vi "DAQ.vi"() -> ()   [LabVIEW 2018]
uses:
  <vilib>/Simulation/DiscreteLinear/Implementation/NILVSim Discrete Transfer Function Direct.llb/SIM Discrete Transfer Function Diagram (SISO CD).vi
  <vilib>/Simulation/ContinuousLinear/Implementation/Shared/SIM Transfer Function Support.llb/SIM Convert CD TF to SIM (SISO).vi
  <vilib>/Simulation/ContinuousLinear/Implementation/Shared/SIM Transfer Function Support.llb/SIM TransferFunction Normalize to Buffer.vi
  <vilib>/Simulation/DiscreteLinear/Implementation/Shared/SIM Init Discrete States.vi
  <vilib>/Simulation/DiscreteLinear/Implementation/NILVSim Discrete Transfer Function Direct.llb/SIM Transfer Function Direct core (SISO).vi
  <vilib>/Simulation/ContinuousLinear/Implementation/Shared/SIM Transfer Function Support.llb/SIM TransferFunction Normalize.vi
  <vilib>/Simulation/Implementation/Shared/SIM Polynomials.llb/SIM Remove Zero Coefficients (DBL).vi
  <vilib>/addons/Control Design/_Model Construction/Model Creation.llb/Model Creation SubVI/cd_Create Transfer Function Model.vi
  <vilib>/addons/Control Design/_Time Response Analysis/Time Response.llb/Time Response subVI/cd_Step Response (Transfer Function).vi
  <vilib>/addons/Control Design/_Utility/Model Viewer.llb/Model Viewer SubVI/cd_Draw Transfer Function Equation (TF).vi
  <vilib>/addons/Control Design/_Model Conversions/Continuous and Discrete.llb/Continuous and Discrete SubVI/cd_Convert Continuous to Discrete (TF).vi
  <vilib>/Simulation/Implementation/Shared/SIM Polynomials.llb/SIM Divide Polynomials (DBL).vi
  <vilib>/Simulation/Implementation/Shared/SIM BuildSimErr.vi
  <vilib>/addons/control/pid/pid.llb/PID (DBL).vi
  <vilib>/Simulation/Implementation/XNodeFramework/SimXNode/SimX.xnode
  <vilib>/addons/Control Design/_Model Construction/Model Typedefs.llb/CD Transfer Function Model (MIMO).ctl
  <vilib>/addons/Control Design/_Model Construction/Model Typedefs.llb/CD General Elements.ctl
  <vilib>/addons/Control Design/_Model Construction/Model Typedefs.llb/CD Transfer Function Model (SISO).ctl
  <vilib>/addons/Control Design/_Model Conversions/NI_CD_Continuous and Discrete.lvlib
  <vilib>/addons/Control Design/_Model Construction/NI_LinSys_Model Typedefs.lvlib
  <vilib>/addons/control/pid/NI_PID_pid.lvlib
  <vilib>/addons/Control Design/_Model Construction/NI_LinSys_Model Creation.lvlib
  <vilib>/addons/Control Design/_Utility/NI_CD_Model Viewer.lvlib
  <vilib>/addons/Control Design/_Time Response Analysis/NI_CD_Time Response.lvlib
  <vilib>/Analysis/NI_AALPro.lvlib
panel:
  in  "Plant Control":i32(knob) scale=0.0..1.0
  out "Step Response\nGraph":cluster{"time":dbl[], dbl[]}[](graph)
  out "Transfer Function Equation":picture
  in  "Sampling\nTime":dbl
  in  "Blower Opening Control at Plant":dbl(slide) scale=15.0..90.0
  out "Polynomial Fit (Fixed)\nfor Temp-Voltage":i32=2
  in  "Voltage input":dbl(knob) scale=0.0..10.0
  in  "Set Temperature\n Auto Mode":i32(slide) scale=20.0..90.0
  in  "output range":cluster{"output high":dbl, "output low":dbl}
  out "Set Temperature Value":dbl
  in  "PID Gains":T1={"proportional gain (Kc)"=1.0, "integral time (Ti, min)"=0.01, "derivative time (Td, min)"=0.0} {"derivative time (Td, min)" format="%.3f"; "integral time (Ti, min)" format="%.3f"; "proportional gain (Kc)" format="%.3f"}
  out "Voltage vs Time":dbl(graph)
  out "Temperature vs Time":dbl(graph)
  in  "STOP":bool
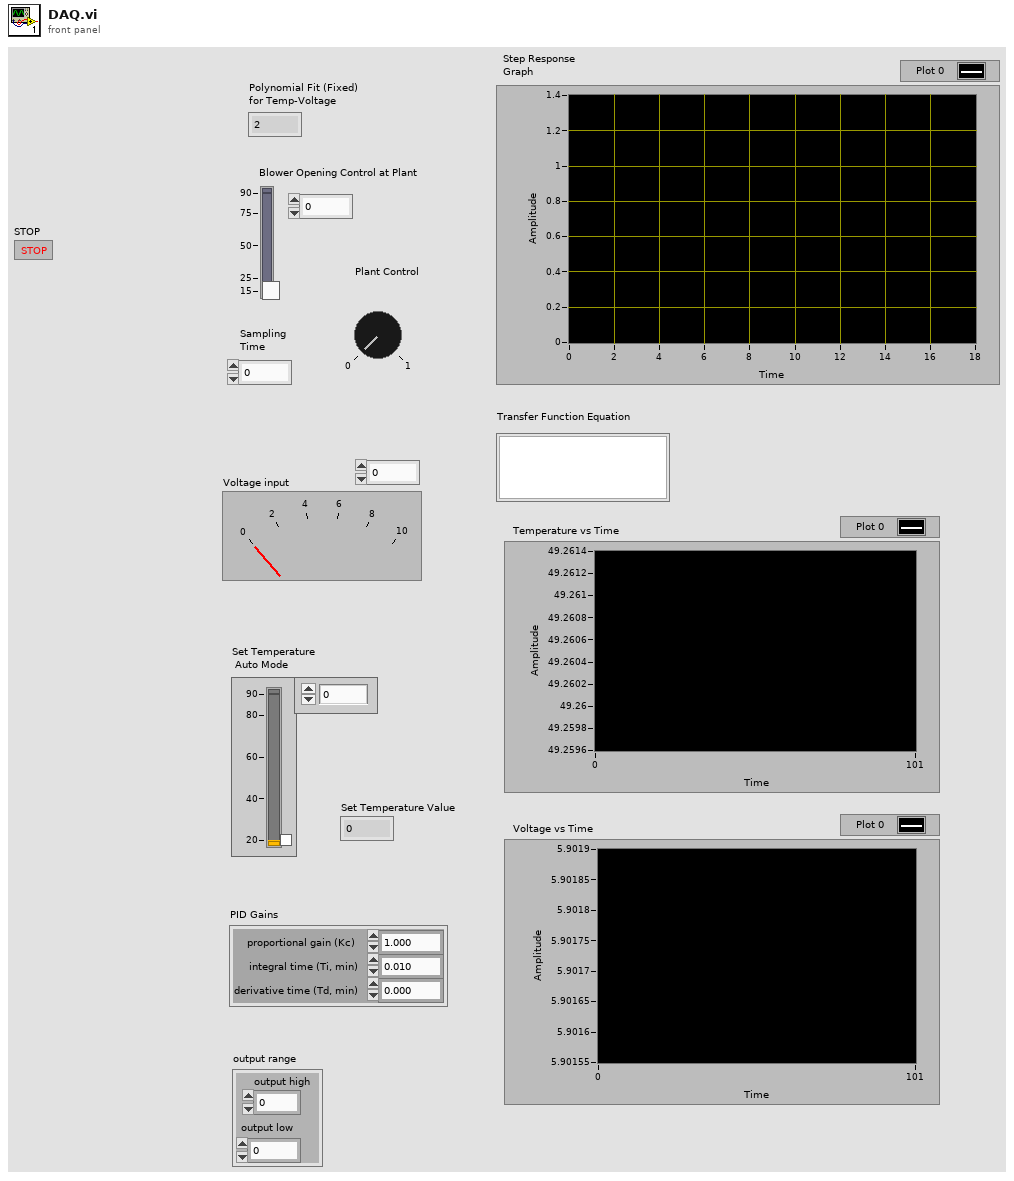
[diagram p1: front panel]
types:
  T1 = cluster{"proportional gain (Kc)":dbl, "integral time (Ti, min)":dbl, "derivative time (Td, min)":dbl}
  T2 = typedef "NI_LinSys_Model Typedefs.lvlib/CD Transfer Function Model (MIMO).ctl" = cluster{"properties":T3, "transfer function(s)":T4[][]}
  T3 = typedef "NI_LinSys_Model Typedefs.lvlib/CD General Elements.ctl" = cluster{"Model name":string, "Input names":string[], "Output names":string[], "Input Delays":dbl[], "Output Delays":dbl[], "Sampling Time":dbl, "Notes":string}
  T4 = typedef "NI_LinSys_Model Typedefs.lvlib/CD Transfer Function Model (SISO).ctl" = cluster{"Numerator":dbl[], "Denominator":dbl[], "delay":dbl}
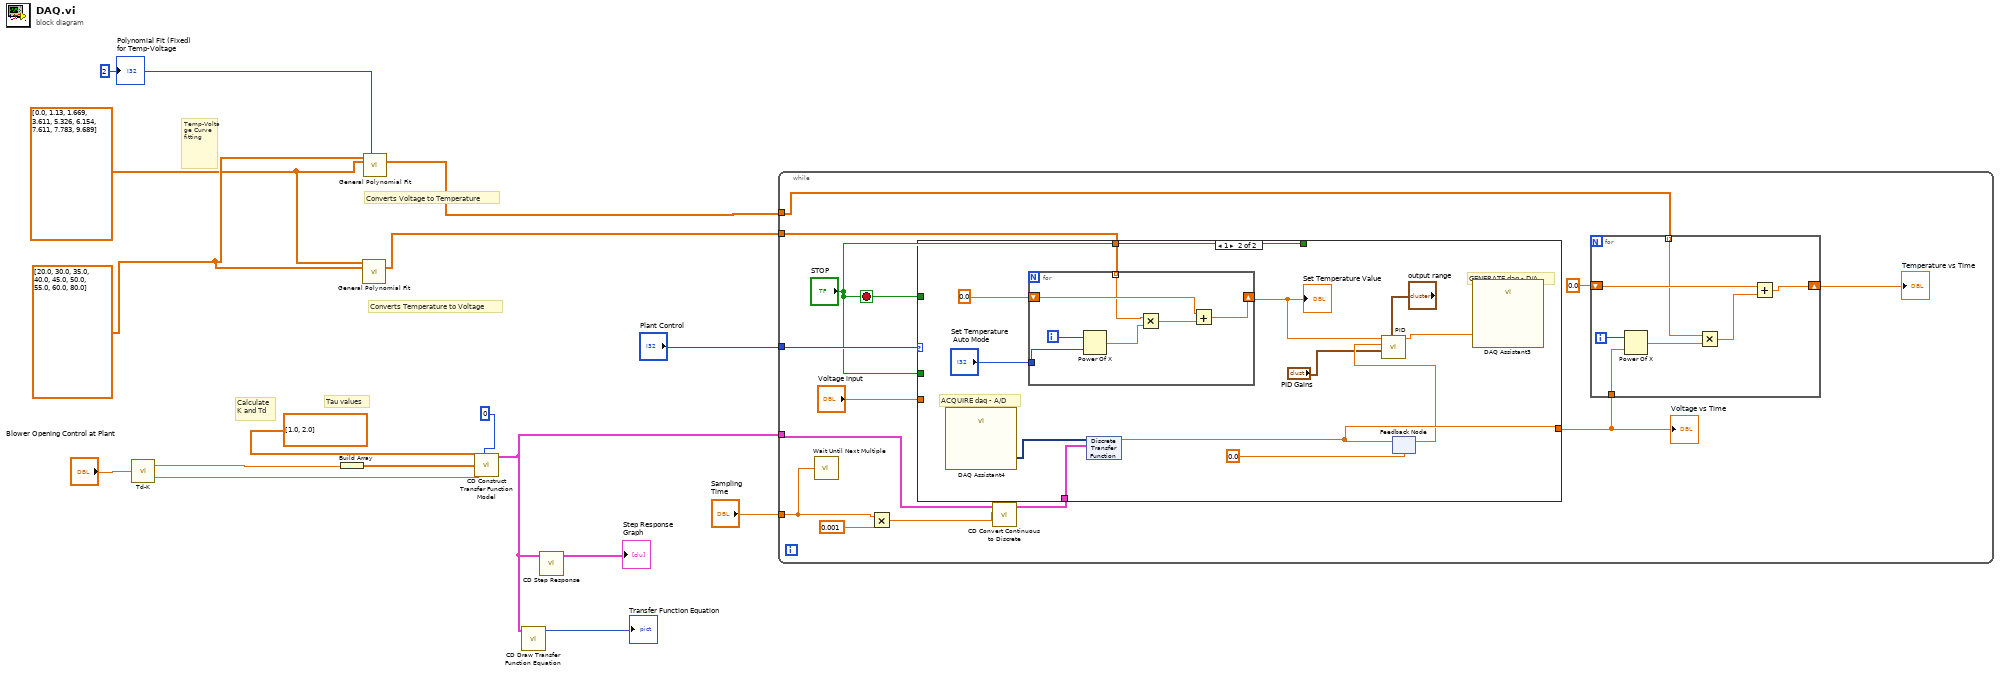
[diagram p0: block diagram]
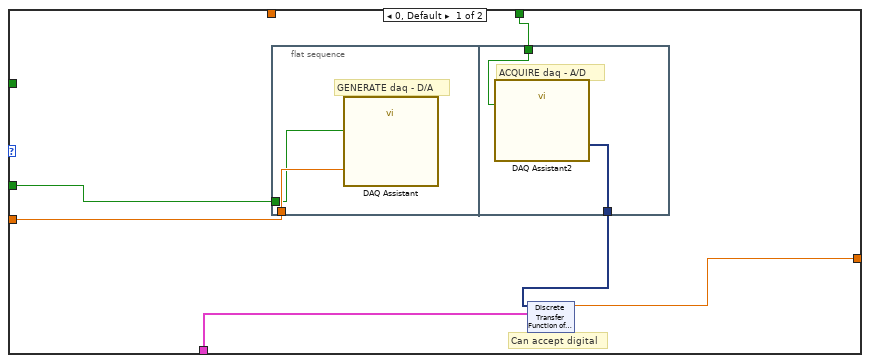
[diagram p2: hidden frame]
diagram:
  w4 = 2
  w2 = dbl[] [0.0, 1.13, 1.669, 3.611, 5.326, 6.154, 7.611, 7.783, 9.689]
  w3 = dbl[] [20.0, 30.0, 35.0, 40.0, 45.0, 50.0, 55.0, 60.0, 80.0]
  # "Converts Voltage to Temperature"
  # "Converts Temperature to Voltage"
  # "Tau values"
  # "Calculate\nK and Td"
  # "Temp-Voltage Curve fitting"
  n1 = call "Td-K.vi"("Blower Opening \nInput (Degrees)"="Blower Opening Control at Plant") -> ("K Calculated"=w14:dbl, "Tau-d Calculated"=w15:dbl)
  n2 = Build Array(w14) -> (w13:dbl[])
  n3 = call <vilib>:"General Polynomial Fit.vi"("Y"=w2, "X"=w3) -> ("Polynomial Coefficients"=w1:dbl[])  [unwired: 10 in, 3 out]
  n4 = call <vilib>:"General Polynomial Fit.vi"("Y"=w3, "polynomial order"=w4, "X"=w2) -> ("Polynomial Coefficients"=w5:dbl[])  [unwired: 9 in, 3 out]
  n5 = call-poly <vilib>:"CD Construct Transfer Function Model.vi"("Sampling Time (s)"=0, "Delay"=w15, "Denominator"=dbl[] [1.0, 2.0], "Numerator"=w13) -> ("Transfer Function Model"=w9:T2)  [unwired: 6 in, 1 out]
  n6 = call-poly <vilib>:"CD Draw Transfer Function Equation.vi"("Transfer Function Model"=w9) -> ("Equation"=→"Transfer Function Equation":picture)  [unwired: 8 in, 2 out]
  n7 = call-poly <vilib>:"CD Step Response.vi"("Transfer Function Model"=w9) -> ("Step Response Graph"=→"Step Response\nGraph":cluster{"time":dbl[], dbl[]}[])  [unwired: 8 in, 2 out]
  n8 = while {
    tunnel: w9 -> [w22]
    tunnel: "Plant Control" -> [w21]
    tunnel: w5 -> [w19]
    tunnel: "Sampling\nTime" -> [w20]
    tunnel: w1 -> [w18]
    stop <- "STOP" stop-if-true
    n9 = call "Wait Until Next Multiple"("Count(mSec)"=w20) -> ()  [unwired: 1 out]
    n10 = Multiply(x=w20, y=0.001) -> (x*y=w28:dbl)
    n11 = call-poly <vilib>:"CD Convert Continuous to Discrete.vi"("Sampling Time (s)"=w28, "Continuous Transfer Function Model"=w22) -> ("Discrete Transfer Function Model"=w26:T2)  [unwired: 8 in, 1 out]
    n12 = case shown="1" w21 {
      tunnel: "Voltage input" -> [w38 _]
      tunnel: "STOP" -> [_ _]
      tunnel: [w41 w59] -> w25
      tunnel: w26 -> [w42 w58]
      tunnel: w18 -> [_ w55]
      tunnel: "STOP" -> [w40 _]
      tunnel: "STOP" -> [w39 _]
      frame 0, Default {
        # "Can accept digital"
        n13 = flat-sequence {
          tunnel: w40 -> [w43]
          tunnel: w38 -> [w44]
          tunnel: w39 -> [w45]
          tunnel: [w46] -> w37
          frame #0 {
            # "GENERATE daq - D/A"
            n14 = call "DAQ Assistant"("data"=w44, "stop (T)"=w43) -> ()  [unwired: 16 in, 2 out]
          }
          frame #1 {
            # "ACQUIRE daq - A/D"
            n15 = call "DAQ Assistant2"("stop (T)"=w45) -> ("data"=w46:dynamicdata)  [unwired: 16 in, 2 out]
          }
        }
        n16 = xnode "Discrete Transfer \nFunction of plant"("input u(k)"=w37, "Transfer Function"=w42) -> ("output y(k)"=w41:dbl)  [unwired: 2 in, 1 out]
      }
      frame 1 {
        # "ACQUIRE daq - A/D"
        # "GENERATE daq - D/A"
        n17 = call "DAQ Assistant4"() -> ("data"=w54:dynamicdata)  [unwired: 17 in, 2 out]
        n18 = for {
          shift-right: [w67] -> w62
          shift-left: 0.0 -> [w66]
          tunnel: "Set Temperature\n Auto Mode" -> [w71]
          tunnel: w55 -> [w65] mode=indexing
          i -> [w70]
          n19 = Power Of X(1:w71, 2:w70) -> (0:w69:dbl)
          n20 = Multiply(x=w65, y=w69) -> (x*y=w68:dbl)
          n21 = Add(x=w66, y=w68) -> (x+y=w67:dbl)
        }
        "Set Temperature Value" <- w62
        n22 = xnode "Discrete Transfer Function"("input u(k)"=w54, "Transfer Function"=w58) -> ("output y(k)"=w59:dbl)  [unwired: 2 in, 1 out]
        n23 = feedback-in #1(w59) -> ()
        n24 = feedback #1(0.0) -> (w57:dbl)
        n25 = call-poly <vilib>:"PID.vi"("output range"="output range", "PID gains"="PID Gains", "process variable"=w57, "setpoint"=w62) -> ("output"=w53:dbl)  [unwired: 6 in, 1 out]
        n26 = call "DAQ Assistant3"("data"=w53) -> ()  [unwired: 17 in, 2 out]
      }
    }
    "Voltage vs Time" <- w25
    n27 = for {
      shift-right: [w31] -> w23
      shift-left: 0.0 -> [w34]
      tunnel: w25 -> [w36]
      tunnel: w19 -> [w30] mode=indexing
      i -> [w35]
      n28 = Power Of X(1:w36, 2:w35) -> (0:w33:dbl)
      n29 = Multiply(x=w30, y=w33) -> (x*y=w32:dbl)
      n30 = Add(x=w34, y=w32) -> (x+y=w31:dbl)
    }
    "Temperature vs Time" <- w23
  }
  "Polynomial Fit (Fixed)\nfor Temp-Voltage" <- w4
